vi "IL Turbo Valve.vi"(4 "Add to (Deny)":T1, 5 "Ignore (F)":bool, 6 "Interlock Condition (ON/OFF)":bool=TRUE, 7 "Stop Self on IL? (T)":bool=TRUE, 8 "error in (no error)":errorcluster, 11 "Interlock Chain in":refnum<class "Interlock Chain.lvclass">) -> (0 "error out":errorcluster, 2 "IL Turbo Valve":refnum<class "Interlock.lvclass">, 3 "Interlock Chain out":refnum<class "Interlock Chain.lvclass">)   [LabVIEW 2015, in "cRIO-Carbondioxide.lvlib" / "cRIO-CO2.lvlib" / "cRIO-CO2.lvclass"]
uses:
  cRIO-CO2.lvclass
  Interlocks/Interlock Chain/Interlock Chain.lvclass
  Interlocks/Controls/Add IL to -Enumerator.ctl
  Interlocks/Interlock/Interlock.lvclass
  Interlocks/Interlock Bool/Interlock Bool.lvclass
  Interlocks/Interlock Bool/Interlock Bool.lvclass/Interlock Bool.ctl
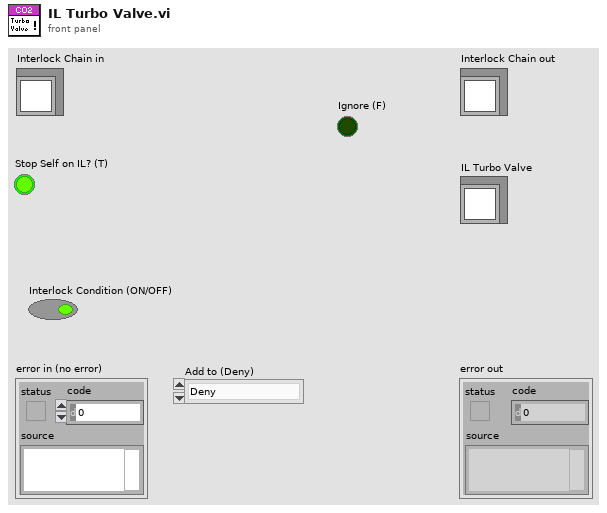
[diagram p1: front panel]
types:
  T1 = typedef "Add IL to -Enumerator.ctl" = enum16{"Deny", "Allow", "None"}
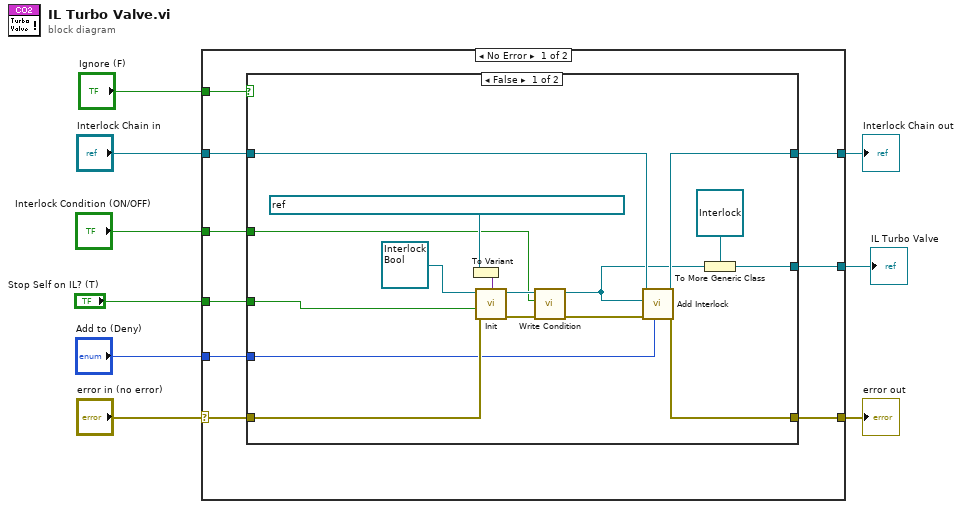
[diagram p0: block diagram]
diagram:
  n1 = case shown="No Error" "error in (no error)" {
    selector: "error in (no error)" -> [w15 w38]
    tunnel: [w14 w38] -> w8
    tunnel: [w16 w37] -> w6
    tunnel: "Interlock Chain in" -> [w17 w37]
    tunnel: "Interlock Condition (ON/OFF)" -> [w18 _]
    tunnel: "Add to (Deny)" -> [w13 _]
    tunnel: [w12 _] -> w3
    tunnel: "Stop Self on IL? (T)" -> [w11 _]
    tunnel: "Ignore (F)" -> [w10 _]
    frame No Error {
      n2 = case shown="False" w10 {
        tunnel: w18 -> [w30 _]
        tunnel: w17 -> [w28 w36]
        tunnel: [w27 w36] -> w16
        tunnel: w15 -> [w26 w35]
        tunnel: [w25 w35] -> w14
        tunnel: w13 -> [w24 _]
        tunnel: [w22 _] -> w12
        tunnel: w11 -> [w19 _]
        frame False {
          n3 = To Variant(anything=refnum<k21> "ni.var.psp://10.2.0.20/AMS Gas SHV/Valves/Turbo Valve" ("SHV")) -> (Variant=w20:variant)
          n4 = call-dynamic "Init.vi"("SHV"=w20, "error in (no error)"=w26, "Stop Self on IL? (T)"=w19, "Interlock in"=refnum<class "Interlock Bool.lvclass"> refnum ("Interlock Bool.lvclass")) -> ("error out"=w31:errorcluster, "Interlock out"=w32:refnum<class "Interlock Bool.lvclass">)  [unwired: 6 in]
          n5 = call "Write Condition.vi"("error in (no error)"=w31, "Interlock Condition"=w30, "Interlock Bool in"=w32) -> ("error out"=w29:errorcluster, "Interlock Bool out"=w23:refnum<class "Interlock Bool.lvclass">)  [unwired: 7 in]
          n6 = call "Add Interlock.vi"("Add to (Deny)"=w24, "error in (no error)"=w29, "Interlock.lvclass"=w23, "Interlock Chain in"=w28) -> ("error out"=w25:errorcluster, "Interlock Chain out"=w27:refnum<class "Interlock Chain.lvclass">)  [unwired: 6 in]
          n7 = To More Generic Class(target class=refnum<class "Interlock.lvclass"> refnum ("Interlock.lvclass"), reference=w23) -> (generic class reference=w22:refnum<class "Interlock.lvclass">)
        }
        frame True {
        }
      }
    }
    frame Error {
    }
  }
  "error out" <- w8
  "Interlock Chain out" <- w6
  "IL Turbo Valve" <- w3
